vi "Initialize.vi"(8 "error in":errorcluster, 9 "Number of Channels":u32=1, 10 "Plugin Name":string, 11 "Voltage Control in":refnum<class "Voltage Control.lvclass">) -> (0 "error out":errorcluster, 3 "Voltage Control out":refnum<class "Voltage Control.lvclass">)   [LabVIEW 2023, in "Voltage Control.lvclass"]
uses:
  Voltage Control.lvclass
  Voltage Control.lvclass/Voltage Control.ctl
  <vilib>/ADAS Replay HIL/Channels/Tag Wrapper/Polymorphic/Open Consumer Tag (Double).vi
  <vilib>/ADAS Replay HIL/Channels/Tag Wrapper/Polymorphic/Open Consumer Tag (Double).vi/bacb721e-673a-491a-accd-959f2e1f334e.vi
  <vilib>/ADAS Replay HIL/Channels/Tag Wrapper/Polymorphic/Open Consumer Tag (Double).vi/bacb721e-673a-491a-accd-959f2e1f334e.vi/c28b0ead-42ad-4072-80a2-aca7f2bd7ce3.vi
  <vilib>/ADAS Replay HIL/AdasHilServices/AdasHilServices Fill In Error Info Ex.vi
  <vilib>/ADAS Replay HIL/Channels/Tag Wrapper/Tag Wrapper.lvlib
  Utilities/Utilities.lvlib
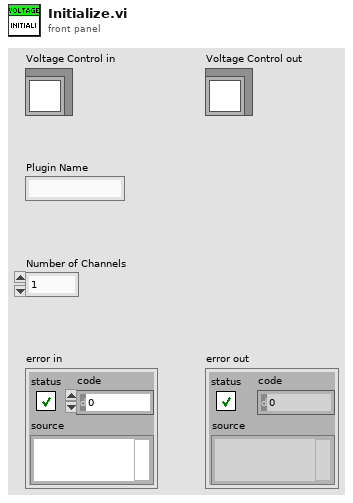
[diagram p1: front panel]
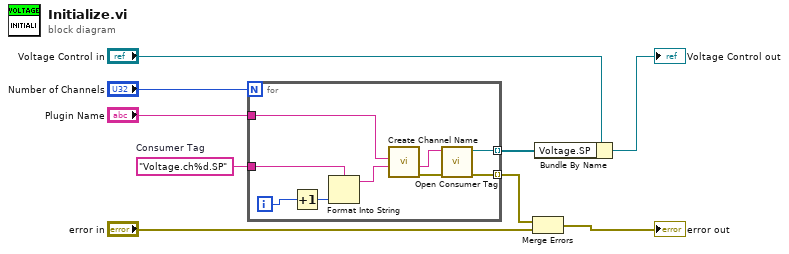
[diagram p0: block diagram]
diagram:
  w9 = "Voltage.ch%d.SP"  # Consumer Tag
  n1 = for {
    N: "Number of Channels" -> [_]
    tunnel: w9 -> [w10]
    tunnel: "Plugin Name" -> [w17]
    tunnel: [w15] -> w5 mode=indexing
    tunnel: [w14] -> w2 mode=indexing
    i -> [w12]
    n2 = Increment(x=w12) -> (x+1=w11:i32)
    n3 = Format Into String(format string=w10, w11) -> (resulting string=w13:string)  [unwired: 2 in, 1 out]
    n4 = call "Create Channel Name.vi"("Channel Name"=w13, "Plugin Name"=w17) -> ("error out"=w16:errorcluster, "Data Channel Name"=w18:string)  [unwired: 8 in]
    n5 = call-poly <vilib>:"Open Consumer Tag.vi"("error in"=w16, "Channel Name"=w18) -> ("error out"=w15:errorcluster, "ADAS HIL Channel"=w14:refnum<k21>)  [unwired: 8 in]
  }
  n6 = Merge Errors(w5, "error in") -> (→"error out":errorcluster)
  n7 = Bundle By Name(cluster="Voltage Control in", "Voltage.SP"=w2) -> (→"Voltage Control out":refnum<class "Voltage Control.lvclass">)
